vi "PID转换.vi"(1 "P":dbl min=0.0 format="%.1g", 2 "I":dbl min=0.0 format="%.1g", 3 "D":dbl min=0.0 format="%.1g") -> (8 "PID":string)   [LabVIEW 2016]
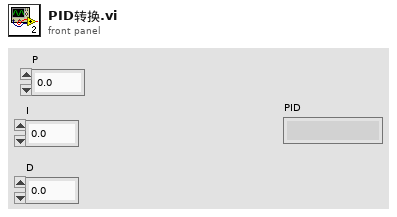
[diagram p1: front panel]
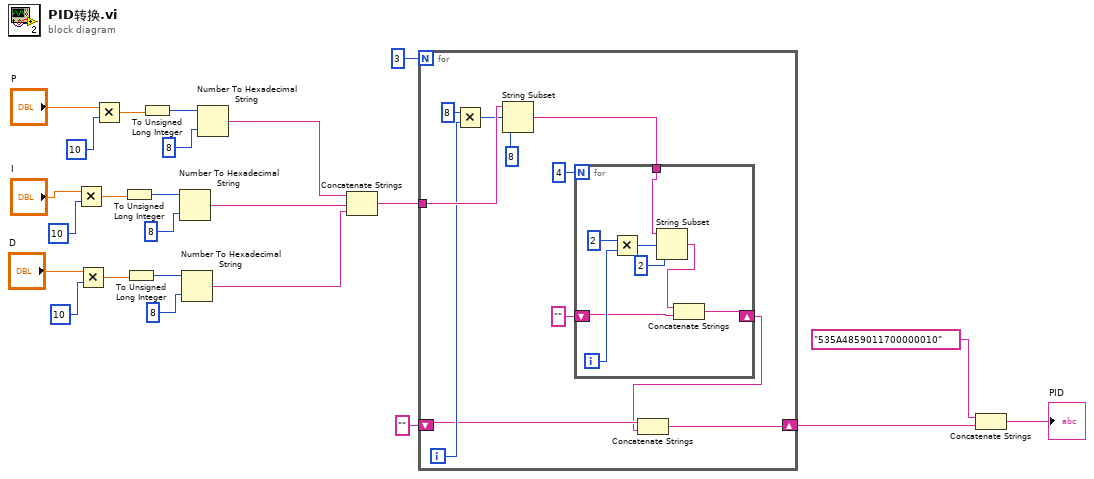
[diagram p0: block diagram]
diagram:
  n1 = Multiply(x="I", y=10) -> (x*y=w17:dbl)
  n2 = Multiply(x="D", y=10) -> (x*y=w13:dbl)
  n3 = Multiply(x="P", y=10) -> (x*y=w21:dbl)
  n4 = To Unsigned Long Integer(number=w17) -> (unsigned 32bit integer=w16:u32)
  n5 = To Unsigned Long Integer(number=w13) -> (unsigned 32bit integer=w12:u32)
  n6 = To Unsigned Long Integer(number=w21) -> (unsigned 32bit integer=w20:u32)
  n7 = Number To Hexadecimal String(1:8, 2:w16) -> (0:w8:string)
  n8 = Number To Hexadecimal String(1:8, 2:w12) -> (0:w7:string)
  n9 = Number To Hexadecimal String(1:8, 2:w20) -> (0:w9:string)
  n10 = Concatenate Strings(w9, w8, w7) -> (w6:string)
  n11 = for {
    N: 3 -> [_]
    tunnel: w6 -> [w34]
    shift-right: [w26] -> w3
    shift-left: "" -> [w27]
    i -> [w31]
    n12 = Multiply(x=u8 8, y=w31) -> (x*y=w33:i32)
    n13 = String Subset(string=w34, offset (0)=w33, length (rest)=8 ("长度（剩余）")) -> (substring=w29:string)
    n14 = for {
      N: 4 -> [_]
      tunnel: w29 -> [w43]
      shift-right: [w37] -> w25
      shift-left: "" -> [w38]
      i -> [w41]
      n15 = Multiply(x=2, y=w41) -> (x*y=w42:i32)
      n16 = String Subset(string=w43, offset (0)=w42, length (rest)=2 ("长度（剩余）")) -> (substring=w36:string)
      n17 = Concatenate Strings(w36, w38) -> (w37:string)
    }
    n18 = Concatenate Strings(w27, w25) -> (w26:string)
  }
  n19 = Concatenate Strings("535A4859011700000010", w3) -> (→"PID":string)
